vi "OAT Orbit Plot.vi"   [LabVIEW 2017]
doc: "Draws an orbit plot on an XY graph. You can use this polymorphic VI to draw an orbit plot with unfiltered or filtered data. Unfiltered data comes from the <B>even angle signals</B> input, filtered data from the <B>magnitudes</B> and <B>phases [phase lag]</B> inputs. The data type you wire to the <B>even angle signals</B> input determines the polymorphic instance to use."
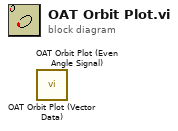
[diagram p0: block diagram]
diagram:
  n1 = call <vilib>:"OAT Orbit Plot (Vector Data).vi"() -> ()  [unwired: 13 in, 3 out]
  n2 = call <vilib>:"OAT Orbit Plot (Even Angle Signal).vi"() -> ()  [unwired: 14 in, 2 out]
